vi "Music Library To Album Library Display.vi"(8 "error in (no error)":errorcluster, 11 "MusicLibrary":refnum<class "MusicLibrary.lvclass">) -> (0 "error out":errorcluster, 3 "Music Library Display Array":T1[](array[typedef]) {"Duration (s)" format="%<%M:%S>T"})   [LabVIEW 2015, in "SongBrowserActor.lvlib" / "SongBrowserActor.lvclass"]
uses:
  SongBrowserActor.lvclass
  controls/Music Library Element Display.ctl
  file/MusicElement/Song/Song Duration.ctl
  file/MusicElement/MusicElementLibrary/MusicLibrary/MusicLibrary.lvclass
  file/MusicElement/MusicElementLibrary/MusicElementLibrary.lvclass/MusicElementLibrary.ctl
  file/MusicElement/Album/Album.lvclass
  file/MusicElement/Album/Album.lvclass/Album.ctl
  file/MusicElement/MusicElement.lvclass/MusicElement.ctl
  file/MusicElement/MusicElementLibrary/Read Music Element Library.vi
  file/MusicElement/MusicElement.lvclass
  file/MusicElement/MusicElementLibrary/SongLibrary/SongLibrary.lvclass
  file/MusicElement/Song/Song.lvclass
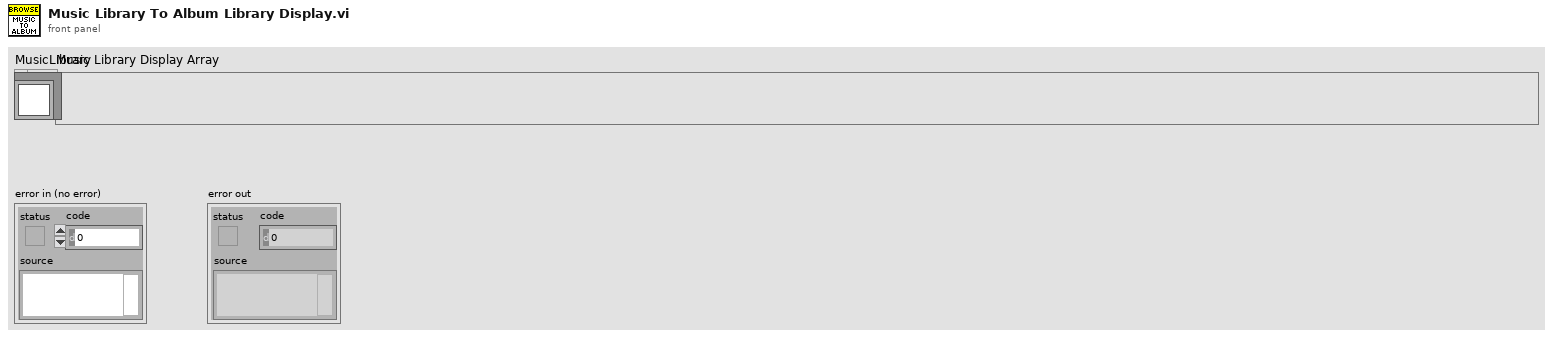
[diagram p1: front panel]
types:
  T1 = typedef "Music Library Element Display.ctl" = cluster{"Name":string, "Details":string, "Duration (s)":T2, "Click":bool}
  T2 = typedef "Song.lvclass/Song Duration.ctl" = timestamp
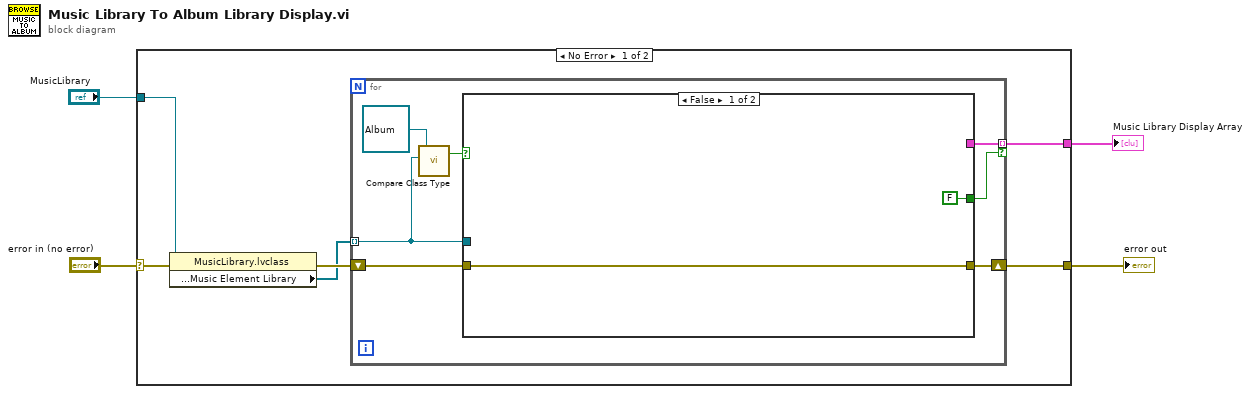
[diagram p0: block diagram]
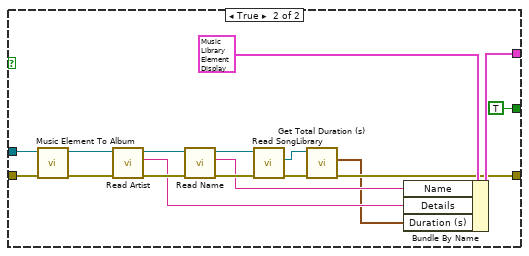
[diagram p2: hidden frame]
diagram:
  n1 = case shown="No Error" "error in (no error)" {
    selector: "error in (no error)" -> [w10 w37]
    tunnel: [w6 w37] -> w3
    tunnel: "MusicLibrary" -> [w9 _]
    tunnel: [w5 _] -> w2
    frame No Error {
      n2 = property class="MusicLibrary.lvclass"(reference=w9, error in=w10) -> (error out=w8:errorcluster, "Data Member Accessors:Music Element Library"=w7:refnum<class "MusicElement.lvclass">[])  [unwired: 1 out]
      n3 = for {
        shift-right: [w16] -> w6
        shift-left: w8 -> [w12]
        tunnel: w7 -> [w11] mode=indexing
        tunnel: [w17] -> w5 mode=indexing if=w15
        n4 = call "Compare Class Type.vi"("MusicElement Check"=w11, "MusicElement in"=refnum<class "Album.lvclass"> refnum ("Album")) -> ("Same Class Type?"=w14:bool)  [unwired: 3 in]
        n5 = case shown="False" w14 {
          tunnel: [_ w36] -> w17
          tunnel: [w18 w26] -> w16
          tunnel: [FALSE TRUE] -> w15
          tunnel: w12 -> [w18 w23]
          tunnel: w11 -> [_ w21]
          frame False {
          }
          frame True {
            n6 = call "Music Element To Album.vi"("error in (no error)"=w23, "MusicElement"=w21) -> ("error out"=w22:errorcluster, "Album"=w20:refnum<class "Album.lvclass">)  [unwired: 8 in]
            n7 = call "Read Artist.vi"("error in (no error)"=w22, "Album in"=w20) -> ("error out"=w30:errorcluster, "Artist"=w28:string, "Album out"=w31:refnum<class "Album.lvclass">)  [unwired: 7 in]
            n8 = call "Read Name.vi"("error in (no error)"=w30, "MusicElement in"=w31) -> ("error out"=w32:errorcluster, "Name"=w29:string, "MusicElement out"=w33:refnum<class "Album.lvclass">)  [unwired: 7 in]
            n9 = call "Read SongLibrary.vi"("error in (no error)"=w32, "Album in"=w33) -> ("error out"=w27:errorcluster, "SongLibrary.lvclass"=w34:refnum<class "SongLibrary.lvclass">)  [unwired: 7 in, 1 out]
            n10 = call "Get Total Duration (s).vi"("error in (no error)"=w27, "SongLibrary in"=w34) -> ("error out"=w26:errorcluster, "Duration (s)"=w25:T2)  [unwired: 7 in, 1 out]
            n11 = Bundle By Name(cluster=T1 {"Name"="", "Details"="", "Duration (s)"=timestamp(0 s since 1904-01-01), "Click"=FALSE} ("Element"), "Name"=w29, "Details"=w28, "Duration (s)"=w25) -> (w36:T1)
          }
        }
      }
    }
    frame Error {
    }
  }
  "error out" <- w3
  "Music Library Display Array" <- w2
